vi "Sub_volage_read_begin.vi"() -> (0 "error out":errorcluster, 1 "data":dbl[](array[numeric]), 3 "Task out":refnum<k21>, 4 "relative seconds":dbl)   [LabVIEW 2021]
uses:
  <vilib>/DAQmx/read.llb/DAQmx Read (Analog 1D DBL 1Chan NSamp).vi
  <vilib>/DAQmx/create/channels.llb/DAQmx Create Channel (AI-Voltage-Basic).vi
  <vilib>/DAQmx/configure/timing.llb/DAQmx Timing (Sample Clock).vi
  <vilib>/DAQmx/miscellaneous.llb/DAQmx Fill In Error Info.vi
panel:
  out "rate":dbl
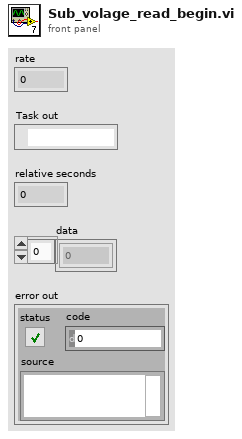
[diagram p1: front panel]
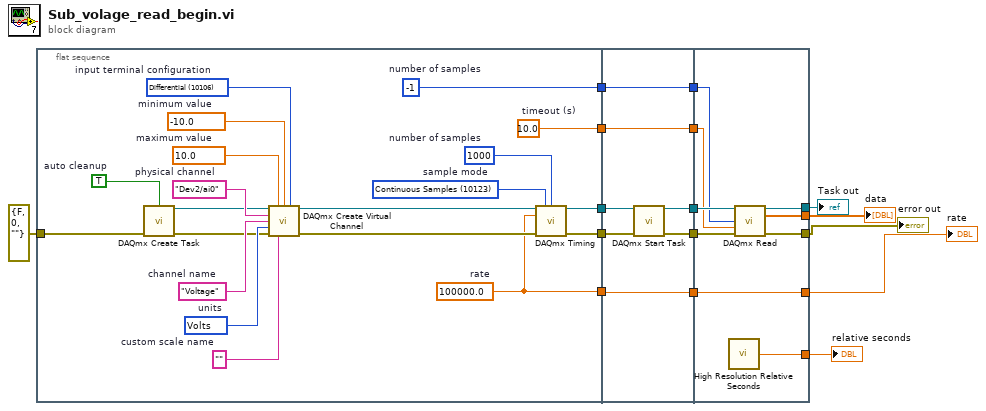
[diagram p0: block diagram]
diagram:
  n1 = flat-sequence {
    tunnel: [w33] -> w16
    tunnel: [w32] -> w15
    tunnel: errorcluster {"status"=FALSE, "code"=0, "source"=""} ("error in") -> [w20]
    tunnel: [w19] -> w14
    tunnel: [w18] -> w13
    tunnel: [w17] -> w3
    tunnel: w16 -> [w42]
    tunnel: w15 -> [w43]
    tunnel: w14 -> [w39]
    tunnel: w13 -> [w40]
    tunnel: [w41] -> w12
    tunnel: [w40] -> w11
    tunnel: [w39] -> w10
    tunnel: [w38] -> w9
    tunnel: w3 -> [w37]
    tunnel: [w37] -> w2
    tunnel: [w46] -> w4
    tunnel: [w47] -> w6
    tunnel: [w48] -> w5
    tunnel: w12 -> [w52]
    tunnel: w11 -> [w51]
    tunnel: w10 -> [w50]
    tunnel: w9 -> [w49]
    tunnel: [w45] -> w7
    tunnel: [w44] -> w1
    tunnel: w2 -> [w44]
    frame #0 {
      w19 = 10.0  # timeout (s)
      w18 = -1  # number of samples
      w36 = 10123 items=["Finite Samples"=10178, "Continuous Samples"=10123, "Hardware Timed Single Point"=12522]  # sample mode
      w35 = 1000  # number of samples
      w17 = 100000.0  # rate
      w31 = 10106 items=["default"=-1, "RSE"=10083, "NRSE"=10078, "Differential"=10106, "Pseudodifferential"=12529]  # input terminal configuration
      w30 = 10348 items=["Volts"=10348, "From Custom Scale"=10065]  # units
      w29 = "Voltage"  # channel name
      w27 = ""  # custom scale name
      w26 = -10.0  # minimum value
      w25 = 10.0  # maximum value
      w24 = "Dev2/ai0"  # physical channel
      w22 = TRUE  # auto cleanup
      n2 = call <vilib>:"DAQmx Create Task.vi"("auto cleanup"=w22, "error in"=w20) -> ("task out"=w23:refnum<k21>, "error out"=w21:errorcluster)  [unwired: 12 in]
      n3 = call-poly <vilib>:"DAQmx Create Virtual Channel.vi"("task in"=w23, "maximum value"=w25, "minimum value"=w26, "input terminal configuration"=w31, "physical channels"=w24, "name to assign"=w29, "units"=w30, "error in"=w21, "custom scale name"=w27) -> ("task out"=w34:refnum<k21>, "error out"=w28:errorcluster)  [unwired: 5 in]
      n4 = call-poly <vilib>:"DAQmx Timing.vi"("task/channels in"=w34, "sample mode"=w36, "samples per channel"=w35, "rate"=w17, "error in"=w28) -> ("task out"=w32:refnum<k21>, "error out"=w33:errorcluster)  [unwired: 9 in]
    }
    frame #1 {
      n5 = call <vilib>:"DAQmx Start Task.vi"("task/channels in"=w43, "error in"=w42) -> ("task out"=w41:refnum<k21>, "error out"=w38:errorcluster)  [unwired: 12 in]
    }
    frame #2 {
      n6 = call <vilib>:"High Resolution Relative Seconds.vi"() -> ("relative seconds"=w45:dbl)
      n7 = call-poly <vilib>:"DAQmx Read.vi"("task/channels in"=w52, "number of samples per channel"=w51, "timeout"=w50, "error in"=w49) -> ("task out"=w48:refnum<k21>, "data"=w47:dbl[], "error out"=w46:errorcluster)  [unwired: 9 in]
    }
  }
  "relative seconds" <- w7
  "rate" <- w1
  "data" <- w6
  "error out" <- w4
  "Task out" <- w5
